vi "Compile Recursivly.vi"(8 "error in (no error)":errorcluster, 9 "Message Priority":T1=enum."Normal", 10 "Override Look up table":variant, 11 "Uncompiled sequence in":T4[](array[typedef])) -> (0 "error out":errorcluster, 1 "Success?":bool, 2 "Override Data":T2[](array[typedef]), 3 "Compiled Message Array":refnum<class "Message.lvclass">[](array[class]))   [LabVIEW 2020, in "Sequencer.lvlib"]
doc: "Recusivly compile an uncompiled sequence into a message array."
uses:
  Sequencer.lvlib
  Controls/Ctl_SequenceElement.ctl
  Controls/Ctl_SequenceControlElement.ctl
  PPL/HDH.Actor Framework.Core.Msg.lvlibp/Flex Msg/Controls/Ctl_Control Element.ctl
  PPL/HDH.Actor Framework.Core.Actor.lvlibp/1abvi3w/vi.lib/ActorFramework/Message/Message.lvclass
  Controls/Ctl_FlexDataElements.ctl
  Controls/Ctl_FlexDataElement.ctl
  PPL/HDH.Actor Framework.Core.Actor.lvlibp/1abvi3w/vi.lib/ActorFramework/Message Enqueuer/Message Priority.ctl
  PPL/HDH.Actor Framework.Core.Msg.lvlibp/Flex Msg/Flex Msg.lvclass
  C:/Current projects/WS/PPL/HDH.Actor Framework.Core.Actor.lvlibp/1abvi3w/vi.lib/ActorFramework/Message/Message.lvclass
  Sequencer Messages/Batch Msg/Batch Msg.lvclass
  C:/Current projects/WS/PPL/HDH.Actor Framework.Core.Msg.lvlibp/Flex Msg/Flex Msg.lvclass
  Sequencer Messages/Loop Msg/Loop Msg.lvclass
  C:/Current projects/WS/HDH.ActorFramework.Core/Actor/Sequencer/Sequencer Messages/Batch Msg/Batch Msg.lvclass
  Sequencer Messages/Batch End Msg/Batch End Msg.lvclass
  Sequencer Messages/Batch Msg/Batch Msg.lvclass/Batch Msg.ctl
  Sequencer Messages/Loop Msg/Loop Msg.lvclass/Loop Msg.ctl
  PPL/HDH.Data.Generic.lvlibp
  PPL/HDH.Actor Framework.Core.Msg.lvlibp
  PPL/HDH.Actor Framework.Core.Actor.lvlibp/1abvi3w/vi.lib/ActorFramework/Message Enqueuer/Message Enqueuer.lvclass
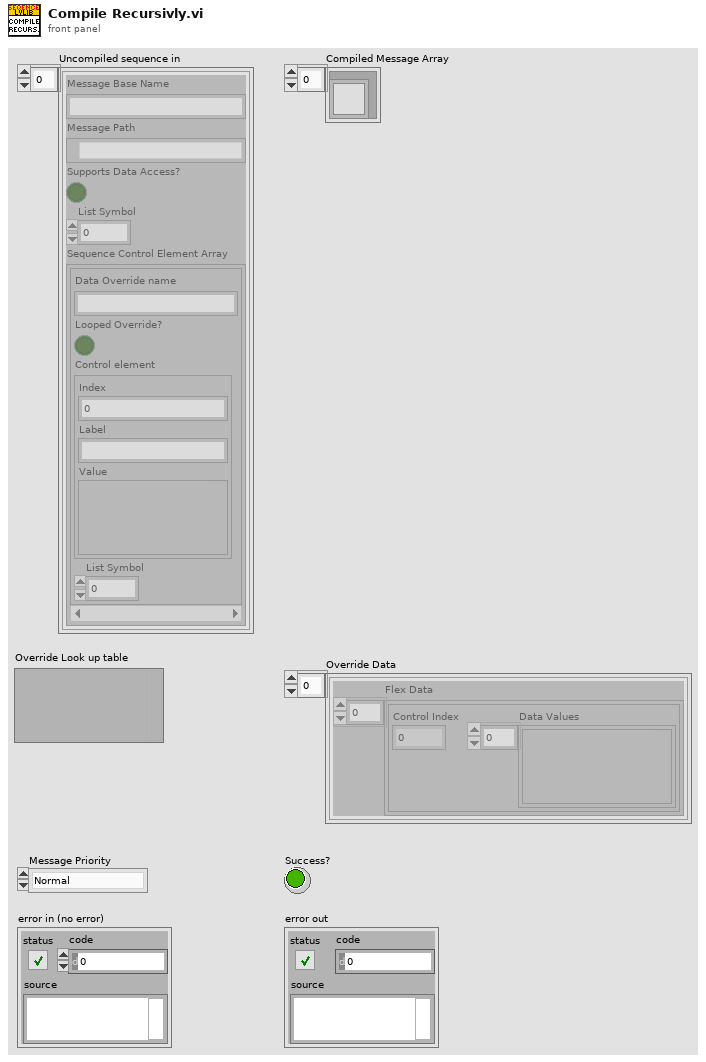
[diagram p1: front panel]
types:
  T1 = typedef "HDH.Actor Framework.Core.Actor.lvlibp/Message Enqueuer.lvclass/Message Priority.ctl" = enum16{"Low", "Normal", "High"}
  T2 = typedef "Sequencer.lvlib/Ctl_FlexDataElements.ctl" = cluster{"Flex Data":T3[]}
  T3 = typedef "Sequencer.lvlib/Ctl_FlexDataElement.ctl" = cluster{"Control Index":i32, "Data Values":variant[]}
  T4 = typedef "Sequencer.lvlib/Ctl_SequenceElement.ctl" = cluster{"Message Base Name":string, "Message Path":path, "Supports Data Access?":bool, "List Symbol":i32, "Sequence Control Element Array":T5[]}
  T5 = typedef "Sequencer.lvlib/Ctl_SequenceControlElement.ctl" = cluster{"Data Override name":string, "Looped Override?":bool, "Control element":T6, "List Symbol":i32}
  T6 = typedef "HDH.Actor Framework.Core.Msg.lvlibp/Ctl_Control Element.ctl" = cluster{"Index":i32, "Label":string, "Value":variant}
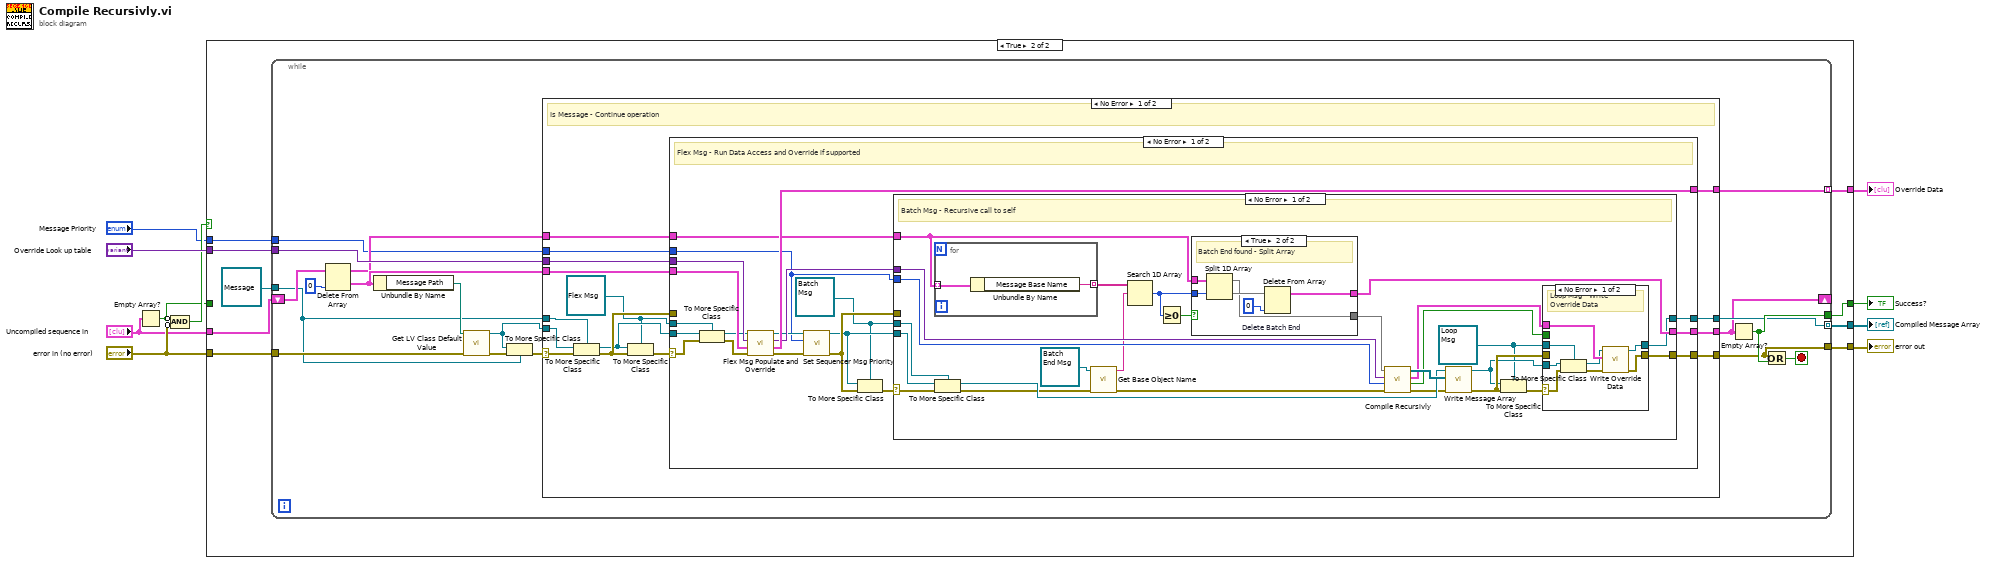
[diagram p0: block diagram]
diagram:
  n1 = Empty Array?(array="Uncompiled sequence in") -> (empty?=w3:bool)
  n2 = Compound Arithmetic op=AND(invert w3, invert "error in (no error)") -> (w5:bool)
  n3 = case shown="True" w5 {
    tunnel: [w12 w15] -> w10
    tunnel: "Uncompiled sequence in" -> [_ w21]
    tunnel: "Override Look up table" -> [_ w17]
    tunnel: [w11 w19] -> w8
    tunnel: [_ w18] -> w7
    tunnel: [_ w16] -> w2
    tunnel: "error in (no error)" -> [w12 w13]
    tunnel: w3 -> [w11 _]
    tunnel: "Message Priority" -> [_ w14]
    frame False {
    }
    frame True {
      n4 = while {
        shift-right: [w25] -> _
        shift-left: w21 -> [w39]
        tunnel: refnum<class "Message.lvclass"> refnum ("Compiled Message Array") -> [w32]
        tunnel: w13 -> [w35]
        tunnel: [w30] -> w19
        tunnel: [w29] -> w18 mode=indexing
        tunnel: w17 -> [w27]
        tunnel: [w24] -> w16 mode=indexing
        tunnel: [w23] -> w15
        tunnel: w14 -> [w22]
        stop <- w33 stop-if-true
        n5 = Delete From Array(array=w39, index=0) -> (deleted portion=w28:T4, array with subset deleted=w26:T4[])  [unwired: 1 in]
        n6 = Unbundle By Name(w28) -> ("Message Path"=w37:path)
        n7 = call <vilib>:"Get LV Class Default Value.vi"("error in (no error)"=w35, "class path"=w37) -> ("error out"=w36:errorcluster, "object"=w31:refnum<class>)  [unwired: 8 in]
        n8 = To More Specific Class(target class=w32, reference=w31, error in=w36) -> (error out=w34:errorcluster)  [unwired: 1 out]
        n9 = case shown="No Error" w34 {
          selector: w34 -> [w54 w128]
          tunnel: [w50 w128] -> w23
          tunnel: w32 -> [w53 w126]
          tunnel: w31 -> [w52 _]
          tunnel: [w48 w126] -> w29
          tunnel: w28 -> [w46 _]
          tunnel: w27 -> [w45 _]
          tunnel: w26 -> [w42 w127]
          tunnel: [w43 w127] -> w25
          tunnel: [w44 _] -> w24
          tunnel: w22 -> [w41 _]
          frame No Error {
            w40 = refnum<class "Flex Msg.lvclass"> refnum ("HDH.Actor Framework.Core.Msg.lvlibp:Flex Msg.lvclass")
            # "Is Message - Continue operation"
            n10 = To More Specific Class(target class=w53, reference=w52, error in=w54) -> (specific class reference=w47:refnum<class "Message.lvclass">, error out=w49:errorcluster)
            n11 = To More Specific Class(target class=w40, reference=w47, error in=w49) -> (error out=w51:errorcluster)  [unwired: 1 out]
            n12 = case shown="No Error" w51 {
              selector: w51 -> [w74 _]
              tunnel: [w61 w125] -> w50
              tunnel: w49 -> [_ w125]
              tunnel: [w62 w124] -> w48
              tunnel: w47 -> [w73 w124]
              tunnel: w40 -> [w72 _]
              tunnel: w46 -> [w71 _]
              tunnel: w45 -> [w70 _]
              tunnel: [w67 _] -> w44
              tunnel: [w63 w123] -> w43
              tunnel: w42 -> [w64 w123]
              tunnel: w41 -> [w56 _]
              frame No Error {
                w55 = refnum<class "Batch Msg.lvclass"> refnum ("Batch Msg")
                # "Flex Msg - Run Data Access and Override if supported"
                n13 = To More Specific Class(target class=w72, reference=w73, error in=w74) -> (specific class reference=w69:refnum<class "Flex Msg.lvclass">, error out=w68:errorcluster)
                n14 = call "Flex Msg Populate and Override.vi"("error in (no error)"=w68, "Sequence Element"=w71, "Override Look up table in"=w70, "Flex Msg in"=w69) -> ("error out"=w60:errorcluster, "Flex Data Elements Cluster Array"=w67:T2, "Override Look up table out"=w65:variant, "Flex Msg out"=w58:refnum<class "Flex Msg.lvclass">)  [unwired: 4 in]
                n15 = call "Set Sequencer Msg Priority.vi"("error in (no error)"=w60, "Message Priority"=w56, "Flex Msg in"=w58) -> ("error out"=w59:errorcluster, "Flex Msg out"=w57:refnum<class "Flex Msg.lvclass">)  [unwired: 7 in]
                n16 = To More Specific Class(target class=w55, reference=w57, error in=w59) -> (error out=w66:errorcluster)  [unwired: 1 out]
                n17 = case shown="No Error" w66 {
                  selector: w66 -> [w98 _]
                  tunnel: w57 -> [w100 w122]
                  tunnel: w55 -> [w99 _]
                  tunnel: [w84 w122] -> w62
                  tunnel: [w93 w121] -> w63
                  tunnel: w64 -> [w95 w121]
                  tunnel: w65 -> [w92 _]
                  tunnel: [w86 w120] -> w61
                  tunnel: w59 -> [_ w120]
                  tunnel: w56 -> [w80 _]
                  frame No Error {
                    w79 = refnum<class "Loop Msg.lvclass"> refnum ("Sequencer.lvlib:Loop Msg.lvclass")
                    # "Batch Msg - Recursive call to self"
                    n18 = for {
                      tunnel: w95 -> [w119] mode=indexing
                      tunnel: [w118] -> w97 mode=indexing
                      n19 = Unbundle By Name(w119) -> ("Message Base Name"=w118:string)
                    }
                    n20 = To More Specific Class(target class=w99, reference=w100, error in=w98) -> (specific class reference=w89:refnum<class "Batch Msg.lvclass">, error out=w76:errorcluster)
                    n21 = call "Get Base Object Name.vi"("error in (no error)"=w76, "Object in"=refnum<class "Batch End Msg.lvclass"> refnum ("Sequencer.lvlib:Batch End Msg.lvclass")) -> ("error out"=w75:errorcluster, "Base class name"=w78:string)  [unwired: 8 in]
                    n22 = Search 1D Array(1D array=w97, element=w78) -> (index of element=w94:i32)  [unwired: 1 in]
                    n23 = Greater Or Equal To 0?(x=w94) -> (x >= 0?=w96:bool)
                    n24 = case shown="True" w96 {
                      tunnel: w95 -> [w111 w117]
                      tunnel: w94 -> [_ w116]
                      tunnel: [_ w113] -> w93
                      tunnel: [w111 w112] -> w91
                      frame False {
                        # "No Batch End - Include all"
                      }
                      frame True {
                        # "Batch End found - Split Array"
                        n25 = Split 1D Array(array=w117, index=w116) -> (first subarray=w112:T4[], second subarray=w115:T4[])
                        n26 = Delete From Array "Delete Batch End"(array=w115, index=0) -> (array with subset deleted=w113:T4[])  [unwired: 1 in, 1 out]
                      }
                    }
                    n27 = call "Compile Recursivly.vi"("error in (no error)"=w75, "Message Priority"=w80, "Override Look up table"=w92, "Uncompiled sequence in"=w91) -> ("error out"=w88:errorcluster, "Success?"=w81:bool, "Override Data"=w82:T2[], "Compiled Message Array"=w90:refnum<class "Message.lvclass">[])  [unwired: 4 in]
                    n28 = call "Write Message Array.vi"("error in (no error)"=w88, "Message Array"=w90, "Batch Msg in"=w89) -> ("error out"=w85:errorcluster, "Batch Msg out"=w83:refnum<class "Batch Msg.lvclass">)  [unwired: 7 in]
                    n29 = To More Specific Class(target class=w79, reference=w83, error in=w85) -> (error out=w87:errorcluster)  [unwired: 1 out]
                    n30 = case shown="No Error" w87 {
                      selector: w87 -> [w108 _]
                      tunnel: [w101 w110] -> w86
                      tunnel: w85 -> [_ w110]
                      tunnel: [w102 w109] -> w84
                      tunnel: w83 -> [w106 w109]
                      tunnel: w79 -> [w107 _]
                      tunnel: w82 -> [w105 _]
                      tunnel: w81 -> [_ _]
                      frame No Error {
                        # "Loop Msg - Write Override Data"
                        n31 = To More Specific Class(target class=w107, reference=w106, error in=w108) -> (specific class reference=w103:refnum<class "Loop Msg.lvclass">, error out=w104:errorcluster)
                        n32 = call "Write Override Data.vi"("error in (no error)"=w104, "Override data"=w105, "Loop Msg in"=w103) -> ("error out"=w101:errorcluster, "Loop Msg out"=w102:refnum<class "Loop Msg.lvclass">)  [unwired: 7 in]
                      }
                      frame Error {
                        # "Not a Loop Msg - No interaction"
                      }
                    }
                  }
                  frame Error {
                    # "Not a Batch Msg - No interaction"
                  }
                }
              }
              frame Error {
                # "Not Flex Msg - No interaction"
              }
            }
          }
          frame Error {
            # "Loading of message failed - Abort"
          }
        }
        n33 = Empty Array?(array=w25) -> (empty?=w30:bool)
        n34 = Or(x=w23, y=w30) -> (x .or. y?=w33:bool)
      }
    }
  }
  "error out" <- w10
  "Compiled Message Array" <- w7
  "Success?" <- w8
  "Override Data" <- w2
